vi "GenerateLab.vi"(8 "ROI":T1={"left"=0, "top"=0, "right"=320, "bottom"=240}, 9 "Lighting":u16(ring)=5 items=["Incandescent/tungsten", "Old direct sunlight at noon", "Old daylight", "ICC profile PCS", "Mid-morning daylight", "Daylight, sRGB, Adobe-RGB", "North sky daylight", "Equal energy", "Daylight Fluorescent", "Cool fluorescent", "White Fluorescent", "Warm White Fluorescent", "Daylight Fluorescent", "Lite White Fluorescent", "Daylight fluorescent, D65 simulator", "Sylvania F40, D50 simulator", "Cool White Fluorescent", "Ultralume 50, Philips TL85", "Ultralume 40, Philips TL84", "Ultralume 30, Philips TL83"], 11 "image data":T2) -> (1 "Dimensions":string, 3 "Plots":T3)   [LabVIEW 2017]
uses:
  <vilib>/picture/picture.llb/imagedata.ctl
panel:
  out "b":dbl[](graph)
  out "a":dbl[](graph)
  out "L":dbl[](graph)
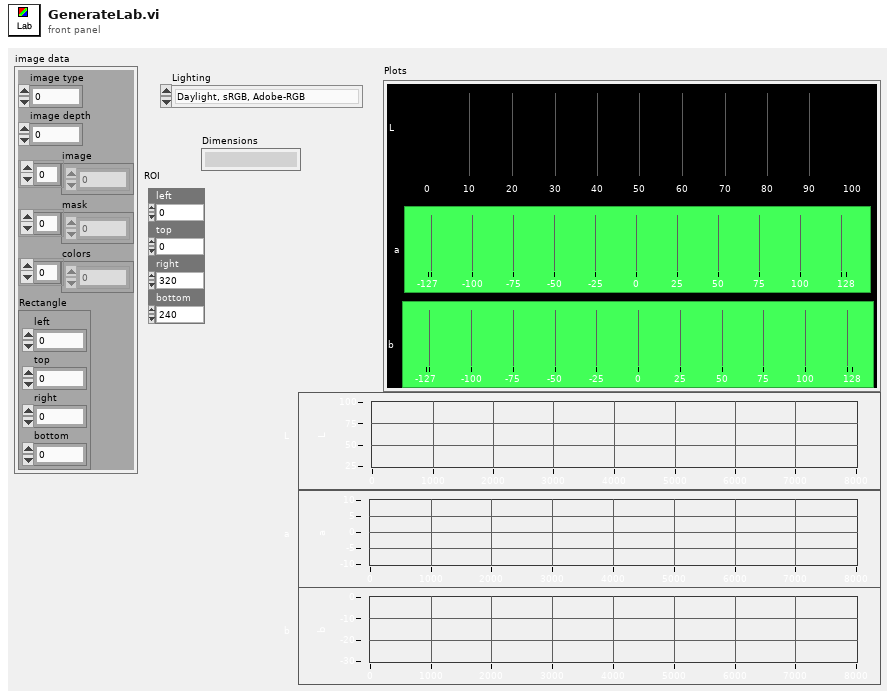
[diagram p1: front panel]
types:
  T1 = cluster{"left":i32, "top":i32, "right":i32, "bottom":i32}
  T2 = typedef "imagedata.ctl" = cluster{"image type":i32, "image depth":i32, "image":u8[], "mask":u8[], "colors":u32[], "Rectangle":cluster{"left":i16, "top":i16, "right":i16, "bottom":i16}}
  T3 = cluster{"L":dbl[], "a":cluster{i32, i32, dbl[]}, "b":cluster{i32, i32, dbl[]}}
  T4 = cluster{dbl[], cluster{i32, i32, dbl[]}, cluster{i32, i32, dbl[]}}
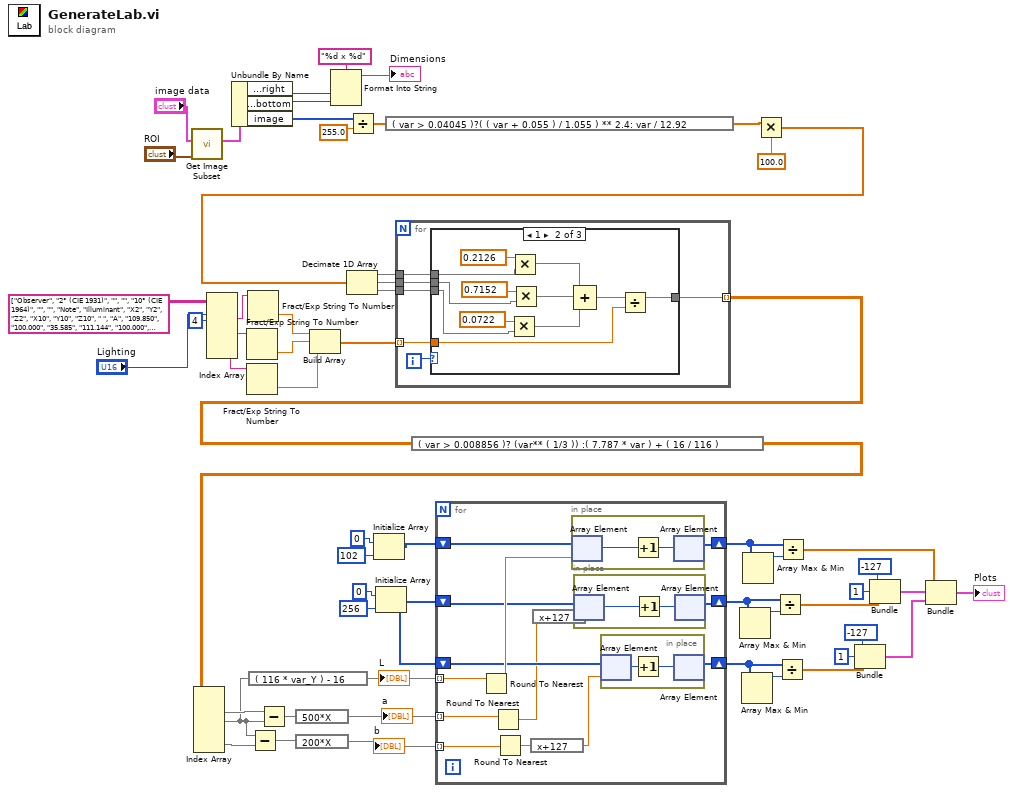
[diagram p0: block diagram]
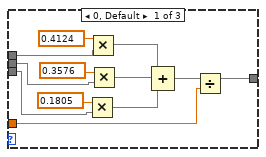
[diagram p2: hidden frame]
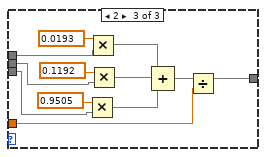
[diagram p3: hidden frame]
diagram:
  n1 = call <vilib>:"Get Image Subset.vi"("subset rect"="ROI", "image data"="image data") -> ("image subset"=w1:T2)  [unwired: 4 in, 1 out]
  n2 = Index Array(array=string[][] [["Observer", "2° (CIE 1931)", "", "", "10° (CIE 1964)", "", "", "Note"], ["Illuminant", "X2", "Y2", "Z2", "X10", "Y10", "Z10", " "], ["A", "109.850", "100.000", "35.585", "111.144", "100.000", "35.200", "Incandescent/tungsten"], ["B", "99.0927", "100.000", "85.313", "99.178;", "100.000", "84.3493", "Old direct sunlight at noon"], ["C", "98.074", "100.000", "118.232", "97.285", "100.000", "116.145", "Old daylight"], ["D50", "96.422", "100.000", "82.521", "96.720", "100.000", "81.427", "ICC profile PCS"], ["D55", "95.682", "100.000", "92.149", "95.799", "100.000", "90.926", "Mid-morning daylight"], ["D65", "95.047", "100.000", "108.883", "94.811", "100.000", "107.304", "Daylight, sRGB, Adobe-RGB"], ["D75", "94.972", "100.000", "122.638", "94.416", "100.000", "120.641", "North sky daylight"], ["E", "100.000", "100.000", "100.000", "100.000", "100.000", "100.000", "Equal energy"], ["F1", "92.834", "100.000", "103.665", "94.791", "100.000", "103.191", "Daylight Fluorescent"], ["F2", "99.187", "100.000", "67.395", "103.280", "100.000", "69.026", "Cool fluorescent"], ["F3", "103.754", "100.000", "49.861", "108.968", "100.000", "51.965", "White Fluorescent"], ["F4", "109.147", "100.000", "38.813", "114.961", "100.000", "40.963", "Warm White Fluorescent"], ["F5", "90.872", "100.000", "98.723", "93.369", "100.000", "98.636", "Daylight Fluorescent"], ["F6", "97.309", "100.000", "60.191", "102.148", "100.000", "62.074", "Lite White Fluorescent"], ["F7", "95.044", "100.000", "108.755", "95.792", "100.000", "107.687", "Daylight fluorescent, D65 simulator"], ["F8", "96.413", "100.000", "82.333", "97.115", "100.000", "81.135", "Sylvania F40, D50 simulator"], ["F9", "100.365", "100.000", "67.868", "102.116", "100.000", "67.826", "Cool White Fluorescent"], ["F10", "96.174", "100.000", "81.712", "99.001", "100.000", "83.134", "Ultralume 50, Philips TL85"], ["F11", "100.966", "100.000", "64.370", "103.866", "100.000", "65.627", "Ultralume 40, Philips TL84"], ["F12", "108.046", "100.000", "39.228", "111.428", "100.000", "40.353", "Ultralume 30, Philips TL83"]] ("Table Control"), index (row) #1="Lighting", index (col) #1=4 ("index (col)")) -> (element #1=w15:string, element #2=w14:string, element #3=w13:string)  [unwired: 4 in]
  n3 = Unbundle By Name(w1) -> ("Rectangle.right"=w19:i16, "Rectangle.bottom"=w18:i16, "image"=w40:u8[])
  n4 = Fract/Exp String To Number(string=w14) -> (number=w9:dbl)  [unwired: 3 in, 1 out]
  n5 = Fract/Exp String To Number(string=w13) -> (number=w8:dbl)  [unwired: 3 in, 1 out]
  n6 = Fract/Exp String To Number(string=w15) -> (number=w10:dbl)  [unwired: 3 in, 1 out]
  n7 = Build Array(w10, w9, w8) -> (w7:dbl[])
  n8 = Format Into String(format string="%d x %d", w19, w18) -> (resulting string=→"Dimensions":string)  [unwired: 2 in, 1 out]
  n9 = Divide(x=w40, y=255.0) -> (x/y=w57:dbl[])
  n10 = Initialize Array(u32 0, 102 ("dimension size")) -> (w37:u32[])
  n11 = Initialize Array(u32 0, 256 ("dimension size")) -> (w44:u32[])
  n12 = expression code="( var > 0.04045 )?( ( var + 0.055 ) / 1.055 ) ** 2.4: var / 12.92"(w57) -> (w42:dbl[])
  n13 = Multiply(x=w42, y=100.0) -> (x*y=w41:dbl[])
  n14 = Decimate 1D Array(w41) -> (w56:dbl[], w55:dbl[], w54:dbl[])
  n15 = for {
    tunnel: w56 -> [w63]
    tunnel: w55 -> [w62]
    tunnel: w54 -> [w61]
    tunnel: [w60] -> w53 mode=indexing
    tunnel: w7 -> [w59] mode=indexing
    i -> [w64]
    n16 = case shown="1" w64 {
      tunnel: w63 -> [w75 w87 w99]
      tunnel: w62 -> [w74 w86 w98]
      tunnel: w61 -> [w73 w85 w97]
      tunnel: [w66 w78 w90] -> w60
      tunnel: w59 -> [w65 w77 w89]
      frame 0, Default {
        n17 = Multiply(x=0.1805, y=w73) -> (x*y=w68:dbl[])
        n18 = Multiply(x=0.4124, y=w75) -> (x*y=w69:dbl[])
        n19 = Multiply(x=0.3576, y=w74) -> (x*y=w70:dbl[])
        n20 = Compound Arithmetic op=ADD(w69, w70, w68) -> (w67:dbl[])
        n21 = Divide(x=w67, y=w65) -> (x/y=w66:dbl[])
      }
      frame 1 {
        n22 = Multiply(x=0.0722, y=w85) -> (x*y=w80:dbl[])
        n23 = Multiply(x=0.2126, y=w87) -> (x*y=w81:dbl[])
        n24 = Multiply(x=0.7152, y=w86) -> (x*y=w82:dbl[])
        n25 = Compound Arithmetic op=ADD(w81, w82, w80) -> (w79:dbl[])
        n26 = Divide(x=w79, y=w77) -> (x/y=w78:dbl[])
      }
      frame 2 {
        n27 = Multiply(x=0.9505, y=w97) -> (x*y=w92:dbl[])
        n28 = Multiply(x=0.0193, y=w99) -> (x*y=w93:dbl[])
        n29 = Multiply(x=0.1192, y=w98) -> (x*y=w94:dbl[])
        n30 = Compound Arithmetic op=ADD(w93, w94, w92) -> (w91:dbl[])
        n31 = Divide(x=w91, y=w89) -> (x/y=w90:dbl[])
      }
    }
  }
  n32 = expression code="( var > 0.008856 )? (var** ( 1/3 )) :( 7.787 * var ) + ( 16 / 116 )"(w53) -> (w52:dbl[][])
  n33 = Index Array(array=w52) -> (element #1=w51:dbl[], element #2=w49:dbl[], element #3=w50:dbl[])  [unwired: 6 in]
  n34 = expression code="( 116 * var_Y ) - 16"(w49) -> (w6:dbl[])
  "L" <- w6
  n35 = Subtract(x=w49, y=w50) -> (x-y=w47:dbl[])
  n36 = Subtract(x=w51, y=w49) -> (x-y=w48:dbl[])
  n37 = expression code="500*X"(w48) -> (w4:dbl[])
  "a" <- w4
  n38 = expression code="200*X"(w47) -> (w5:dbl[])
  "b" <- w5
  n39 = for {
    shift-right: [w112] -> w35
    shift-left: w37 -> [w114]
    shift-right: [w109] -> w33
    shift-left: w44 -> [w110]
    shift-right: [w108] -> w31
    shift-left: w44 -> [w111]
    tunnel: w6 -> [w103] mode=indexing
    tunnel: w4 -> [w102] mode=indexing
    tunnel: w5 -> [w101] mode=indexing
    n40 = Round To Nearest(number=w103) -> (nearest integer value=w113:dbl)
    n41 = Round To Nearest(number=w102) -> (nearest integer value=w106:dbl)
    n42 = Round To Nearest(number=w101) -> (nearest integer value=w107:dbl)
    n43 = expression code="x+127"(w107) -> (w104:dbl)
    n44 = expression code="x+127"(w106) -> (w105:dbl)
    n45 = in-place {
      n46 = in-place-array #1(w114, w113) -> (w120:u32)
      n47 = Increment(x=w120) -> (x+1=w119:u32)
      n48 = in-place-array #1(w119) -> (w112:u32[])  [unwired: 1 out]
    }
    n49 = in-place {
      n50 = in-place-array #2(w110, w105) -> (w118:u32)
      n51 = Increment(x=w118) -> (x+1=w117:u32)
      n52 = in-place-array #2(w117) -> (w109:u32[])  [unwired: 1 out]
    }
    n53 = in-place {
      n54 = in-place-array #3(w111, w104) -> (w116:u32)
      n55 = Increment(x=w116) -> (x+1=w115:u32)
      n56 = in-place-array #3(w115) -> (w108:u32[])  [unwired: 1 out]
    }
  }
  n57 = Array Max & Min(array=w33) -> (max value=w34:u32)  [unwired: 3 out]
  n58 = Array Max & Min(array=w31) -> (max value=w32:u32)  [unwired: 3 out]
  n59 = Array Max & Min(array=w35) -> (max value=w36:u32)  [unwired: 3 out]
  n60 = Divide(x=w33, y=w34) -> (x/y=w30:dbl[])
  n61 = Divide(x=w31, y=w32) -> (x/y=w25:dbl[])
  n62 = Divide(x=w35, y=w36) -> (x/y=w24:dbl[])
  n63 = Bundle(-127, 1, w25) -> (w22:cluster{i32, i32, dbl[]})  [unwired: 1 in]
  n64 = Bundle(-127, 1, w30) -> (w23:cluster{i32, i32, dbl[]})  [unwired: 1 in]
  n65 = Bundle(w24, w23, w22) -> (→"Plots":T4)  [unwired: 1 in]
